vi "Creators Created Events.vi"(8 "Created Event Alias":string, 9 "Priority?":bool, 10 "Msg Strategy":refnum<class "Msg Strategy.lvclass">, 11 "Base Event in":refnum<class "Base Event.lvclass">) -> (3 "Base Event out":refnum<class "Base Event.lvclass">)   [LabVIEW 2021, in "jettl.lvlib" / "Base Event.lvlib" / "Base Event.lvclass"]
uses:
  Base Event.lvclass
  C:/git/jettl/src/jettl/jettl/jettl.lvclass
  Msg Strategy/Msg Strategy.lvclass
  Base Event.lvclass/Base Event.ctl
  Queue Mailbox/Queue Mailbox.lvlib
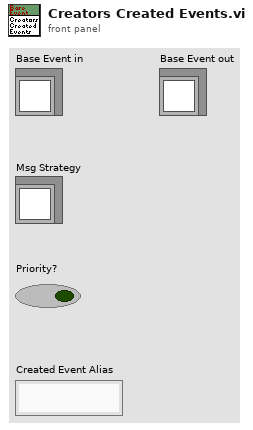
[diagram p1: front panel]
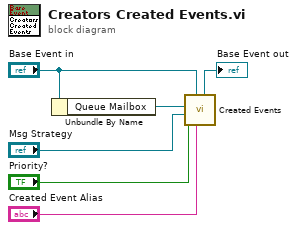
[diagram p0: block diagram]
diagram:
  n1 = Unbundle By Name("Base Event in") -> ("Queue Mailbox"=w6:refnum<data-value>)
  n2 = call "Created Events.vi"("Created Event Alias"="Created Event Alias", "jettl in"="Base Event in", "Priority?"="Priority?", "Msg Strategy"="Msg Strategy", "Queue Mailbox"=w6) -> ("jettl out"=→"Base Event out":refnum<class "Base Event.lvclass">)  [unwired: 6 in]
